vi "Control_stage_event_que.vi"(11 "Stage control":T2={"Up"=FALSE, "Left"=FALSE, "Right"=FALSE, "Down"=FALSE, "Z Down"=FALSE, "Z Up"=FALSE, "X Step Size(um)"=10.0, "Z step size (um)"=10.0, "Y Step Size(um)"=10.0, "Enable x-axis"=TRUE, "Enable y-axis"=TRUE, "Enable z-axis"=TRUE, "Same step size"=TRUE, "Global step size (um)"=10.0, "stop"=FALSE, "Destination"={"X Position"=-23.0, "Y Position"=-18.0, "Z Position"=0.0}, "Move to destination"=FALSE}) -> (10 "Stage position":T1={"X Position"=-23.0, "Y Position"=-18.0, "Z Position"=0.0})   [LabVIEW 2020]
uses:
  typedefs/typedef_stage_control.ctl
  typedefs/typedef_stage_position.ctl
  typedefs/typedef_Z_stack.ctl
  typedefs/Laser_toggles_typedef.ctl
  Global stop DAQ.vi
panel:
  in  "Tab Control":enum32{"Manual setup", "Acquisition", "Debug"}(tab)
  out "FirmwareVersion":string="3.03\r"
  out "Connected":bool=TRUE
  in  "Laser order control":T3={"Laser 488 nm power"=0.0, "Laser 560 nm power"=0.0, "Laser 595 nm power"=0.0, "Laser 642 nm power"=0.0, "Laser 560 order selection"=2, "Laser 595 order selection"=0, "Laser 642 order selection"=0, "Laser 488 order selection"=1} {"Laser 488 order selection" items=["Not active", "1", "2", "3", "4"]; "Laser 642 order selection" items=["Not active", "1", "2", "3", "4"]; "Laser 595 order selection" items=["Not active", "1", "2", "3", "4"]; "Laser 560 order selection" items=["Not active", "1", "2", "3", "4"]; "Laser 642 nm power" min=0.0 max=5.0 scale=0.0..100.0; "Laser 595 nm power" min=0.0 max=5.0 scale=0.0..100.0; "Laser 560 nm power" min=0.0 max=5.0 scale=0.0..100.0; "Laser 488 nm power" min=0.0 max=5.0 scale=0.0..100.0}
  in  "Z-stack":T4={"Acquire Z-stack"=FALSE, "Step size (um)"=0.2, "Number of slices"=10.0, "Progress Bar"=10, "Image acquisition time (ms)"=1000.0, "Flyback time (ms)"=32.0} {"Progress Bar" scale=0.0..100.0}
  in  "Voice coil calibration file":path=path "C:/Users/lpk27/Documents/pan-ASLMsynched/pan-ASLM/Calibration files/newcalibration_voice coil input_25msflyback.txt"
  out "Initial offset between stage and generation":u32
  out "Error out":errorcluster
  out "output cluster":T5
  in  "SPIIPLUSCOM660Lib.IAsyncChannel":refnum<k7>
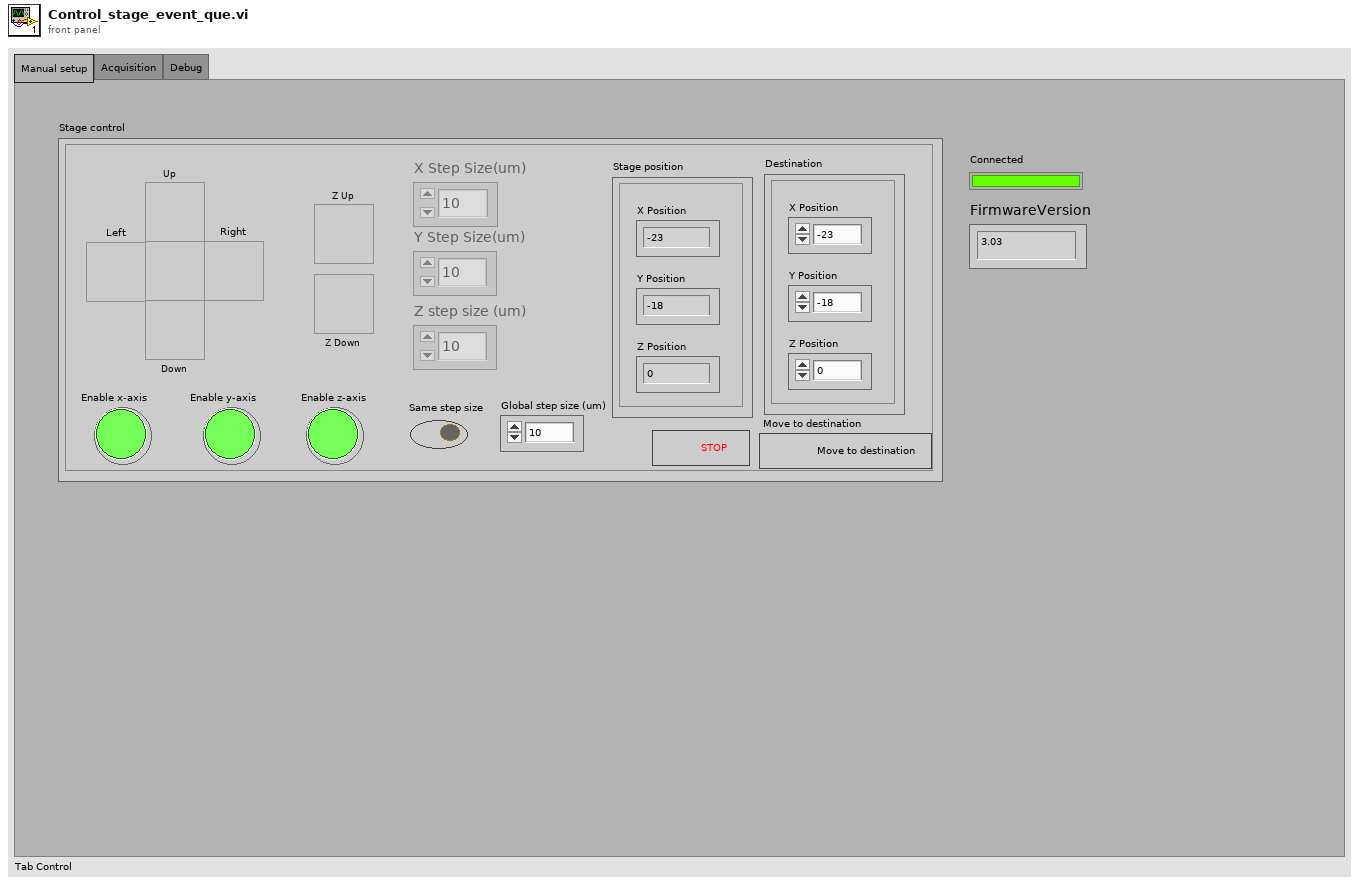
[diagram p1: front panel]
types:
  T1 = typedef "typedef_stage_position.ctl" = cluster{"X Position":dbl, "Y Position":dbl, "Z Position":dbl}
  T2 = typedef "typedef_stage_control.ctl" = cluster{"Up":bool, "Left":bool, "Right":bool, "Down":bool, "Z Down":bool, "Z Up":bool, "X Step Size(um)":dbl, "Z step size (um)":dbl, "Y Step Size(um)":dbl, "Enable x-axis":bool, "Enable y-axis":bool, "Enable z-axis":bool, "Same step size":bool, "Global step size (um)":dbl, "stop":bool, "Destination":T1, "Move to destination":bool}
  T3 = typedef "Laser_toggles_typedef.ctl" = cluster{"Laser 488 nm power":dbl, "Laser 560 nm power":dbl, "Laser 595 nm power":dbl, "Laser 642 nm power":dbl, "Laser 560 order selection":u16, "Laser 595 order selection":u16, "Laser 642 order selection":u16, "Laser 488 order selection":u16}
  T4 = typedef "typedef_Z_stack.ctl" = cluster{"Acquire Z-stack":bool, "Step size (um)":dbl, "Number of slices":dbl, "Progress Bar":u8, "Image acquisition time (ms)":dbl, "Flyback time (ms)":dbl}
  T5 = cluster{"element":string, "reference OUT":refnum<k7>, "error OUT":errorcluster}
  T6 = enum16{"Initialize", "Verify connection", "Running", "Closing"}
  T7 = enum8{"Enabled", "Disabled", "Disabled and Grayed Out"}
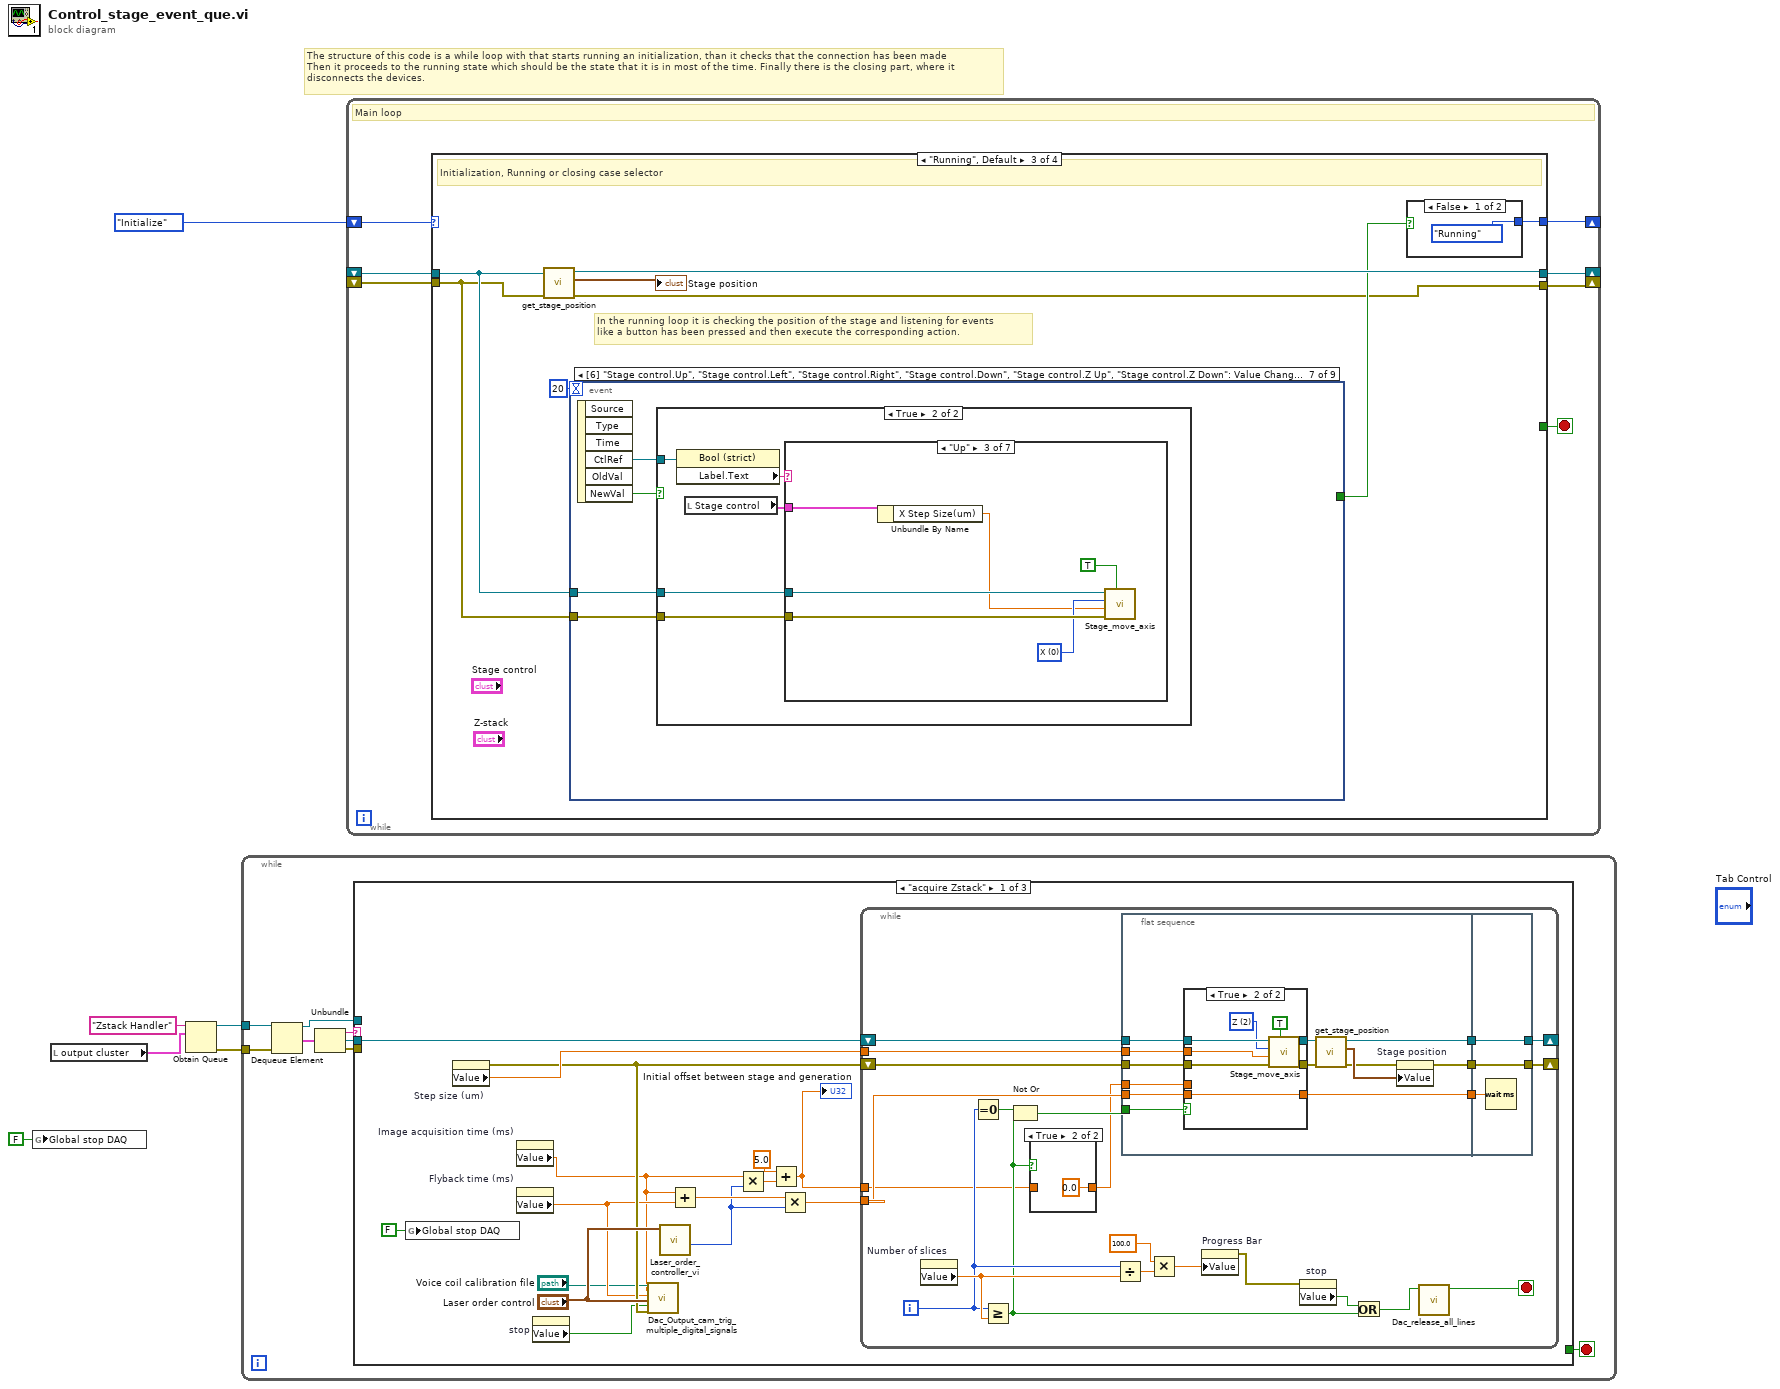
[diagram p0: block diagram]
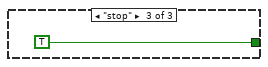
[diagram p5: hidden frame]
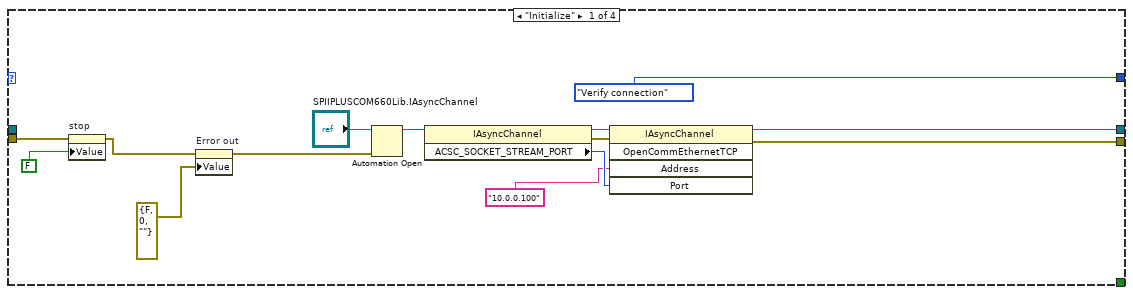
[diagram p6: hidden frame]
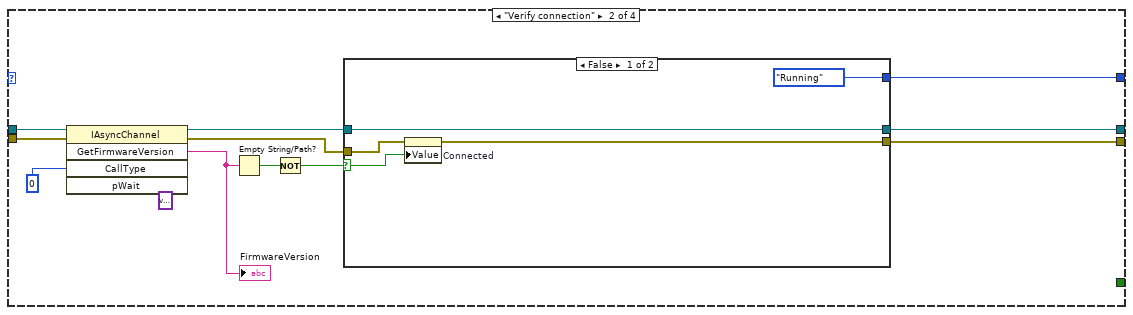
[diagram p7: hidden frame]
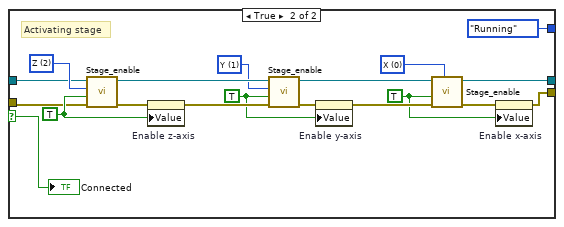
[diagram p8: hidden frame]
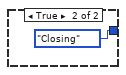
[diagram p9: hidden frame]
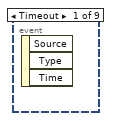
[diagram p10: hidden frame]
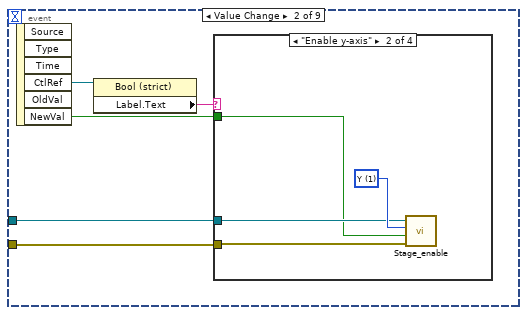
[diagram p11: hidden frame]
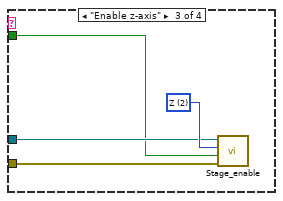
[diagram p13: hidden frame]
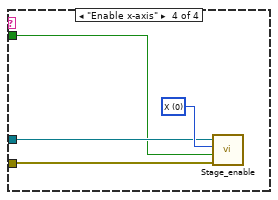
[diagram p14: hidden frame]
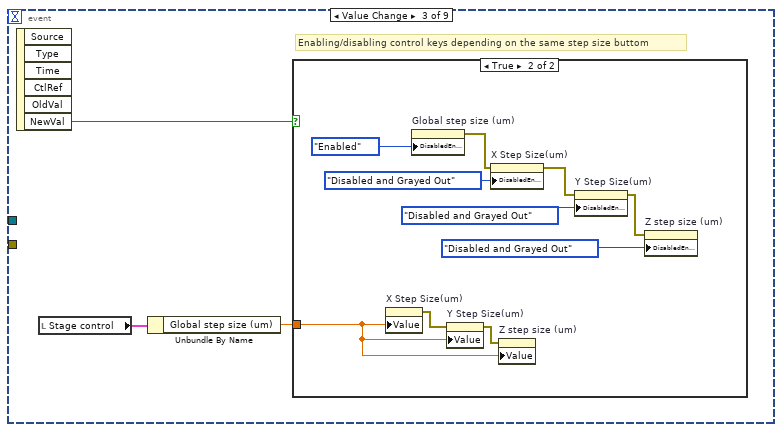
[diagram p15: hidden frame]
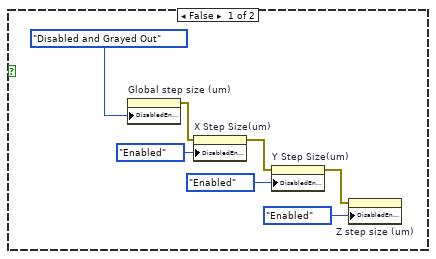
[diagram p16: hidden frame]
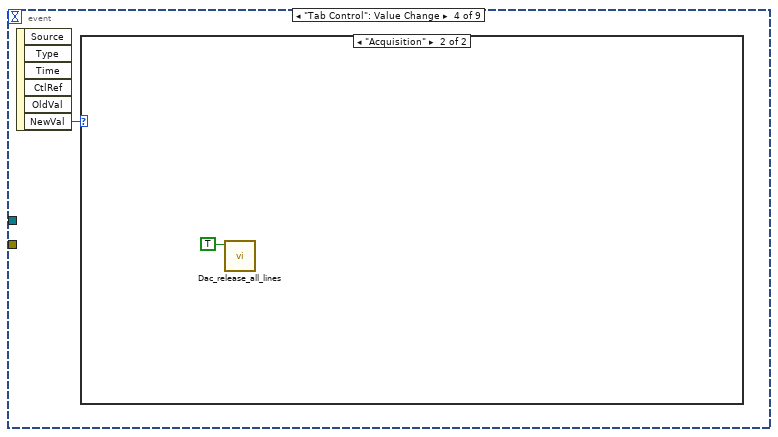
[diagram p17: hidden frame]
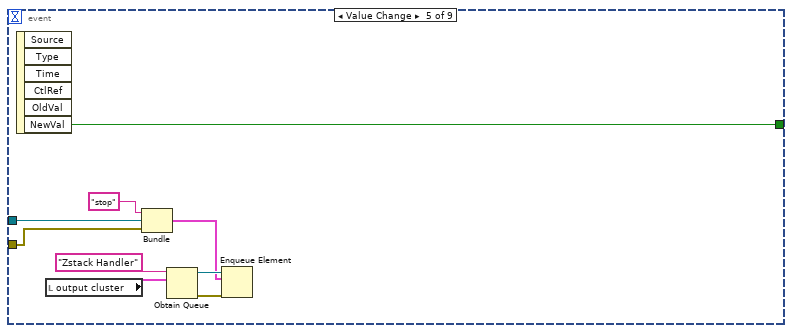
[diagram p19: hidden frame]
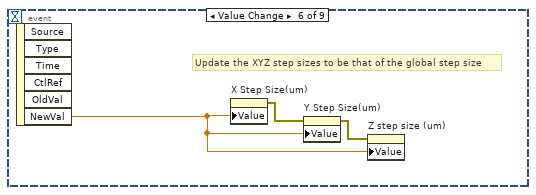
[diagram p20: hidden frame]
diagram:
  # "The structure of this code is a while loop with that starts running an initialization, than it checks that the connection has been made\nThen it proceeds to the running state which should be the state that it is in most of the time. Finally there is the closing part, where it\ndisconnects the devices."
  n1 = global write "Global stop DAQ.vi" "Global stop DAQ"(FALSE ("Global stop DAQ")) -> ()
  n2 = local read "output cluster"() -> (w2:T5)
  n3 = Obtain Queue(name (unnamed)="Zstack Handler", element data type=w2) -> (queue out=w4:refnum<queue>, error out=w3:errorcluster)  [unwired: 3 in, 1 out]
  n4 = while {
    tunnel: w4 -> [w14]
    tunnel: w3 -> [w13]
    stop <- w8 stop-if-true
    n5 = Dequeue Element(queue=w14, error in (no error)=w13) -> (queue out=w7:refnum<queue>, element=w12:T5)  [unwired: 1 in, 2 out]
    n6 = Unbundle(w12) -> ("element"=w11:string, "reference OUT"=w10:refnum<k7>, "error OUT"=w9:errorcluster)
    n7 = case shown="\"acquire Zstack\"" w11 {
      tunnel: w10 -> [w21 _ _]
      tunnel: w9 -> [_ _ _]
      tunnel: [_ _ TRUE] -> w8
      tunnel: w7 -> [_ _ _]
      frame "acquire Zstack" {
        n8 = global write "Global stop DAQ.vi" "Global stop DAQ"(FALSE ("Global stop DAQ")) -> ()
        n9 = property on="Step size (um)" class="DigNum (strict)"() -> (error out=w27:errorcluster, "Value"=w29:dbl)  [unwired: 2 in, 1 out]
        n10 = property on="Image acquisition time (ms)" class="DigNum (strict)"() -> ("Value"=w16:dbl)  [unwired: 2 in, 2 out]
        n11 = property on="Flyback time (ms)" class="DigNum (strict)"() -> ("Value"=w26:dbl)  [unwired: 2 in, 2 out]
        n12 = property on="stop" class="Bool (strict)"() -> ("Value"=w20:bool)  [unwired: 2 in, 2 out]
        n13 = call "Dac_Output_cam_trig_multiple_digital_signals.vi"("File to read"="Voice coil calibration file", "Image acquisition time (ms)"=w16, "Delay between frames"=w26, "Laser Toggles"="Laser order control", "stop"=w20, "error in"=w27) -> ()  [unwired: 13 in, 1 out]
        n14 = call "Laser_order_controller_vi.vi"("Laser Toggles"="Laser order control") -> ("Active lasers"=w18:i16)  [unwired: 8 in, 2 out]
        n15 = Add(x=w16, y=w26) -> (x+y=w25:dbl)
        n16 = Multiply(x=w16, y=w18) -> (x*y=w17:dbl)
        n17 = Add(x=5.0, y=w17) -> (x+y=w15:dbl)
        "Initial offset between stage and generation" <- w15
        n18 = Multiply(x=w25, y=w18) -> (x*y=w23:dbl)
        n19 = while {
          shift-right: [w51] -> _
          shift-left: w21 -> [w52]
          shift-right: [w50] -> _
          shift-left: w27 -> [w38]
          tunnel: w29 -> [w46]
          tunnel: w23 -> [w32]
          tunnel: w15 -> [w31]
          i -> [w37]
          stop <- w41 stop-if-true
          n20 = property on="Number of slices" class="DigNum (strict)"() -> ("Value"=w44:dbl)  [unwired: 2 in, 2 out]
          n21 = Equal To 0?(x=w37) -> (x = 0?=w35:bool)
          n22 = Greater Or Equal?(x=w37, y=w44) -> (x >= y?=w33:bool)
          n23 = Not Or(1:w33, 2:w35) -> (0:w34:bool)
          n24 = case shown="True" w33 {
            tunnel: w31 -> [w53 _]
            tunnel: [w53 0.0] -> w30
            frame False {
            }
            frame True {
            }
          }
          n25 = Divide(x=w37, y=w44) -> (x/y=w48:dbl)
          n26 = flat-sequence {
            tunnel: w52 -> [w67]
            tunnel: w46 -> [w64]
            tunnel: [w66] -> w43
            tunnel: [w65] -> w42
            tunnel: w38 -> [w59]
            tunnel: w34 -> [w58]
            tunnel: w32 -> [w57]
            tunnel: [w56] -> w36
            tunnel: w30 -> [w55]
            tunnel: [w80] -> w50
            tunnel: [w81] -> w51
            tunnel: w43 -> [w81]
            tunnel: w42 -> [w80]
            tunnel: w36 -> [w79]
            frame #0 {
              n27 = case shown="True" w58 {
                tunnel: w67 -> [w70 w78]
                tunnel: w64 -> [_ w77]
                tunnel: [w70 w74] -> w63
                tunnel: [w69 w73] -> w62
                tunnel: w59 -> [w69 w72]
                tunnel: w57 -> [_ w71]
                tunnel: [w68 w71] -> w56
                tunnel: w55 -> [w68 _]
                frame False {
                }
                frame True {
                  w76 = u16 2 items=["X", "Y", "Z"] ("Axes Select")
                  n28 = call "Stage_move_axis.vi"("Direction true means positive increment"=TRUE, "error in (no error)"=w72, "Distance micrometer"=w77, "Axes Select"=w76, "reference IN"=w78) -> ("error OUT"=w73:errorcluster, "reference OUT"=w74:refnum<k7>)  [unwired: 5 in]
                }
              }
              n29 = call "get_stage_position.vi"("error IN"=w62, "reference IN"=w63) -> ("error OUT"=w60:errorcluster, "Stage position OUT"=w61:T1, "reference OUT"=w66:refnum<k7>)  [unwired: 7 in]
              n30 = property on="Stage position" class="Clust (strict)"(error in=w60, "Value"=w61) -> (error out=w65:errorcluster)  [unwired: 1 in, 1 out]
            }
            frame #1 {
              n31 = Wait (ms)(milliseconds to wait=w79) -> ()  [unwired: 1 out]
            }
          }
          n32 = Multiply(x=100.0 ("y"), y=w48) -> (x*y=w45:dbl)
          n33 = property on="Progress Bar" class="Slide (strict)"("Value"=w45) -> (error out=w39:errorcluster)  [unwired: 2 in, 1 out]
          n34 = property on="stop" class="Bool (strict)"(error in=w39) -> ("Value"=w49:bool)  [unwired: 1 in, 2 out]
          n35 = Or(x=w49, y=w33) -> (x .or. y?=w40:bool)
          n36 = call "Dac_release_all_lines.vi"("Release all DAQ lines"=w40) -> ("Finished"=w41:bool)  [unwired: 9 in, 1 out]
        }
      }
      frame Default {
      }
      frame "stop" {
      }
    }
  }
  n37 = while {
    shift-right: [w85] -> _
    shift-left: T6."Initialize" -> [w88]
    shift-right: [w87] -> _
    shift-left: _ -> [w84]
    shift-right: [w86] -> _
    shift-left: _ -> [w83]
    stop <- w89 stop-if-true
    # "Main loop"
    n38 = case shown="\"Running\", Default" w88 {
      tunnel: [_ _ _ TRUE ("NewVal")] -> w89
      tunnel: [w97 w107 w143 _] -> w87
      tunnel: [w96 w105 w140 _] -> w86
      tunnel: [T6."Verify connection" w106 w147 _] -> w85
      tunnel: w84 -> [_ w111 w145 w259]
      tunnel: w83 -> [w93 w110 w144 w258]
      frame "Initialize" {
        n39 = property on="stop" class="Bool (strict)"(error in=w93, "Value"=FALSE) -> (error out=w91:errorcluster)  [unwired: 1 in, 1 out]
        n40 = property on="Error out" class="Clust (strict)"(error in=w91, "Value"=errorcluster {"status"=FALSE, "code"=0, "source"=""} ("Error out")) -> (error out=w90:errorcluster)  [unwired: 1 in, 1 out]
        n41 = Automation Open(error in (no error)=w90, Automation Refnum="SPIIPLUSCOM660Lib.IAsyncChannel") -> (Automation Refnum=w103:refnum<k7>)  [unwired: 2 in, 1 out]
        n42 = property class="IAsyncChannel"(reference=w103) -> (reference out=w102:refnum<k7>, error out=w98:errorcluster, "ACSC_SOCKET_STREAM_PORT"=w100:i32)  [unwired: 1 in]
        n43 = invoke class="IAsyncChannel" method="OpenCommEthernetTCP"(reference=w102, error in=w98, "Address"="10.0.0.100", "Port"=w100) -> (reference out=w97:refnum<k7>, error out=w96:errorcluster)  [unwired: 1 in, 3 out]
      }
      frame "Verify connection" {
        n44 = invoke class="IAsyncChannel" method="GetFirmwareVersion"(reference=w111, error in=w110, "CallType"=u64 0, "pWait"=variant) -> (reference out=w108:refnum<k7>, error out=w104:errorcluster, "GetFirmwareVersion"=w113:string)  [unwired: 1 in, 2 out]
        "FirmwareVersion" <- w113
        n45 = Empty String/Path?(string/path=w113) -> (empty?=w112:bool)
        n46 = Not(x=w112) -> (.not. x?=w109:bool)
        n47 = case shown="False" w109 {
          selector: w109 -> [w120 w139]
          tunnel: w104 -> [w119 w126]
          tunnel: w108 -> [w117 w124]
          tunnel: [w118 w123] -> w105
          tunnel: [w117 w122] -> w107
          tunnel: [T6."Running" T6."Running"] -> w106
          frame False {
            n48 = property on="Connected" class="Bool (strict)"(error in=w119, "Value"=w120) -> (error out=w118:errorcluster)  [unwired: 1 in, 1 out]
          }
          frame True {
            w131 = TRUE ("Boolean")
            w128 = u16 0 items=["X", "Y", "Z"] ("Axes Select")
            w130 = TRUE ("Boolean")
            w127 = u16 1 items=["X", "Y", "Z"] ("Axes Select")
            w129 = TRUE ("Boolean")
            w125 = u16 2 items=["X", "Y", "Z"] ("Axes Select")
            # "Activating stage"
            n49 = call "Stage_enable.vi"("error in (no error)"=w126, "ON=true, OFF = false"=w129, "Axes Select"=w125, "reference"=w124) -> ("error out"=w134:errorcluster, "reference out"=w132:refnum<k7>)  [unwired: 6 in]
            n50 = property on="Enable z-axis" class="Bool (strict)"(error in=w134, "Value"=w129) -> (error out=w135:errorcluster)  [unwired: 1 in, 1 out]
            n51 = call "Stage_enable.vi"("error in (no error)"=w135, "ON=true, OFF = false"=w130, "Axes Select"=w127, "reference"=w132) -> ("error out"=w136:errorcluster, "reference out"=w133:refnum<k7>)  [unwired: 6 in]
            n52 = property on="Enable y-axis" class="Bool (strict)"(error in=w136, "Value"=w130) -> (error out=w137:errorcluster)  [unwired: 1 in, 1 out]
            n53 = call "Stage_enable.vi"("error in (no error)"=w137, "ON=true, OFF = false"=w131, "Axes Select"=w128, "reference"=w133) -> ("error out"=w138:errorcluster, "reference out"=w122:refnum<k7>)  [unwired: 6 in]
            n54 = property on="Enable x-axis" class="Bool (strict)"(error in=w138, "Value"=w131) -> (error out=w123:errorcluster)  [unwired: 1 in, 1 out]
            "Connected" <- w139
          }
        }
      }
      frame "Running", Default {
        # "In the running loop it is checking the position of the stage and listening for events \nlike a button has been pressed and then execute the corresponding action."
        # "Initialization, Running or closing case selector"
        n55 = call "get_stage_position.vi"("error IN"=w144, "reference IN"=w145) -> ("error OUT"=w140:errorcluster, "Stage position OUT"=→"Stage position":T1, "reference OUT"=w143:refnum<k7>)  [unwired: 7 in]
        n56 = event shown="[6] \"Stage control.Up\", \"Stage control.Left\", \"Stage control.Right\", \"Stage control.Down\", \"Stage control.Z Up\", \"Stage control.Z Down\": Value Change" {
          selector: _ -> [_ _ _ _ _ _ _ _ _]
          dyn-events: _ -> [_ _ _ _ _ _ _ _ _]
          timeout: 20 -> [_ _ _ _ _ _ _ _ _]
          tunnel: w145 -> [_ w151 _ _ w191 _ w202 w248 w251]
          tunnel: w144 -> [_ w150 _ _ w190 _ w201 w247 w253]
          tunnel: [_ _ _ _ w197 _ _ _ _] -> w141
          event Timeout {
            n57 = event-data() -> ()  [unwired: 1 in, 3 out]
          }
          event Value Change {
            n58 = event-data() -> ("CtlRef"=w154:refnum<vi>, "NewVal"=w152:bool)  [unwired: 1 in, 4 out]
            n59 = property class="Bool (strict)"(reference=w154) -> ("Label.Text"=w153:string)  [unwired: 1 in, 2 out]
            n60 = case shown="\"Enable y-axis\"" w153 {
              tunnel: w152 -> [_ w155 w159 w163]
              tunnel: w151 -> [_ w156 w161 w165]
              tunnel: w150 -> [_ w157 w160 w164]
              frame Default {
              }
              frame "Enable y-axis" {
                w158 = u16 1 items=["X", "Y", "Z"] ("Axes Select")
                n61 = call "Stage_enable.vi"("error in (no error)"=w157, "ON=true, OFF = false"=w155, "Axes Select"=w158, "reference"=w156) -> ()  [unwired: 6 in, 2 out]
              }
              frame "Enable z-axis" {
                w162 = u16 2 items=["X", "Y", "Z"] ("Axes Select")
                n62 = call "Stage_enable.vi"("error in (no error)"=w160, "ON=true, OFF = false"=w159, "Axes Select"=w162, "reference"=w161) -> ()  [unwired: 6 in, 2 out]
              }
              frame "Enable x-axis" {
                w166 = u16 0 items=["X", "Y", "Z"] ("Axes Select")
                n63 = call "Stage_enable.vi"("error in (no error)"=w164, "ON=true, OFF = false"=w163, "Axes Select"=w166, "reference"=w165) -> ()  [unwired: 6 in, 2 out]
              }
            }
          }
          event Value Change {
            # "Enabling/disabling control keys depending on the same step size buttom"
            n64 = event-data() -> ("NewVal"=w169:bool)  [unwired: 1 in, 5 out]
            n65 = local read "Stage control"() -> (w168:T2)
            n66 = Unbundle By Name(w168) -> ("Global step size (um)"=w167:dbl)
            n67 = case shown="True" w169 {
              tunnel: w167 -> [_ w181]
              frame False {
                n68 = property on="Global step size (um)" class="DigNum (strict)"("DisabledEnum"=T7."Disabled and Grayed Out" ("Disabled")) -> (error out=w170:errorcluster)  [unwired: 2 in, 1 out]
                n69 = property on="X Step Size(um)" class="DigNum (strict)"(error in=w170, "DisabledEnum"=T7."Enabled" ("Disabled")) -> (error out=w174:errorcluster)  [unwired: 1 in, 1 out]
                n70 = property on="Y Step Size(um)" class="DigNum (strict)"(error in=w174, "DisabledEnum"=T7."Enabled" ("Disabled")) -> (error out=w172:errorcluster)  [unwired: 1 in, 1 out]
                n71 = property on="Z step size (um)" class="DigNum (strict)"(error in=w172, "DisabledEnum"=T7."Enabled" ("Disabled")) -> ()  [unwired: 1 in, 2 out]
              }
              frame True {
                n72 = property on="X Step Size(um)" class="DigNum (strict)"("Value"=w181) -> (error out=w180:errorcluster)  [unwired: 2 in, 1 out]
                n73 = property on="Global step size (um)" class="DigNum (strict)"("DisabledEnum"=T7."Enabled" ("Disabled")) -> (error out=w177:errorcluster)  [unwired: 2 in, 1 out]
                n74 = property on="Y Step Size(um)" class="DigNum (strict)"(error in=w180, "Value"=w181) -> (error out=w179:errorcluster)  [unwired: 1 in, 1 out]
                n75 = property on="X Step Size(um)" class="DigNum (strict)"(error in=w177, "DisabledEnum"=T7."Disabled and Grayed Out" ("Disabled")) -> (error out=w184:errorcluster)  [unwired: 1 in, 1 out]
                n76 = property on="Z step size (um)" class="DigNum (strict)"(error in=w179, "Value"=w181) -> ()  [unwired: 1 in, 2 out]
                n77 = property on="Y Step Size(um)" class="DigNum (strict)"(error in=w184, "DisabledEnum"=T7."Disabled and Grayed Out" ("Disabled")) -> (error out=w182:errorcluster)  [unwired: 1 in, 1 out]
                n78 = property on="Z step size (um)" class="DigNum (strict)"(error in=w182, "DisabledEnum"=T7."Disabled and Grayed Out" ("Disabled")) -> ()  [unwired: 1 in, 2 out]
              }
            }
          }
          event "Tab Control": Value Change {
            n79 = event-data() -> ("NewVal"=w187:enum32{"Manual setup", "Acquisition", "Debug"})  [unwired: 1 in, 5 out]
            n80 = case shown="\"Acquisition\"" w187 {
              frame "Manual setup", Default {
              }
              frame "Acquisition" {
                n81 = call "Dac_release_all_lines.vi"("Release all DAQ lines"=TRUE) -> ()  [unwired: 9 in, 2 out]
              }
            }
          }
          event Value Change {
            n82 = event-data() -> ("NewVal"=w197:bool)  [unwired: 1 in, 5 out]
            n83 = local read "output cluster"() -> (w193:T5)
            n84 = Bundle("element"="stop", "reference OUT"=w191, "error OUT"=w190) -> (w189:T5)  [unwired: 1 in]
            n85 = Obtain Queue(name (unnamed)="Zstack Handler", element data type=w193) -> (queue out=w195:refnum<queue>, error out=w194:errorcluster)  [unwired: 3 in, 1 out]
            n86 = Enqueue Element(queue=w195, element=w189, error in (no error)=w194) -> ()  [unwired: 1 in, 3 out]
          }
          event Value Change {
            # "Update the XYZ step sizes to be that of the global step size"
            n87 = event-data() -> ("NewVal"=w200:dbl)  [unwired: 1 in, 5 out]
            n88 = property on="X Step Size(um)" class="DigNum (strict)"("Value"=w200) -> (error out=w199:errorcluster)  [unwired: 2 in, 1 out]
            n89 = property on="Y Step Size(um)" class="DigNum (strict)"(error in=w199, "Value"=w200) -> (error out=w198:errorcluster)  [unwired: 1 in, 1 out]
            n90 = property on="Z step size (um)" class="DigNum (strict)"(error in=w198, "Value"=w200) -> ()  [unwired: 1 in, 2 out]
          }
          event Value Change {
            n91 = event-data() -> ("CtlRef"=w204:refnum<vi>, "NewVal"=w203:bool)  [unwired: 1 in, 4 out]
            n92 = case shown="True" w203 {
              tunnel: w204 -> [_ w209]
              tunnel: w202 -> [_ w206]
              tunnel: w201 -> [_ w205]
              frame False {
              }
              frame True {
                n93 = property class="Bool (strict)"(reference=w209) -> ("Label.Text"=w208:string)  [unwired: 1 in, 2 out]
                n94 = local read "Stage control"() -> (w207:T2)
                n95 = case shown="\"Up\"" w208 {
                  tunnel: w207 -> [w215 w221 w227 w233 w239 w245 _]
                  tunnel: w206 -> [w214 w220 w226 w232 w238 w244 _]
                  tunnel: w205 -> [w213 w219 w225 w231 w237 w243 _]
                  frame "Left" {
                    w211 = u16 1 items=["X", "Y", "Z"] ("Axes Select")
                    n96 = Unbundle By Name(w215) -> ("Y Step Size(um)"=w210:dbl)
                    n97 = call "Stage_move_axis.vi"("Direction true means positive increment"=FALSE, "error in (no error)"=w213, "Distance micrometer"=w210, "Axes Select"=w211, "reference IN"=w214) -> ()  [unwired: 5 in, 2 out]
                  }
                  frame "Right" {
                    w217 = u16 1 items=["X", "Y", "Z"] ("Axes Select")
                    n98 = Unbundle By Name(w221) -> ("Y Step Size(um)"=w216:dbl)
                    n99 = call "Stage_move_axis.vi"("Direction true means positive increment"=TRUE, "error in (no error)"=w219, "Distance micrometer"=w216, "Axes Select"=w217, "reference IN"=w220) -> ()  [unwired: 5 in, 2 out]
                  }
                  frame "Up" {
                    w223 = u16 0 items=["X", "Y", "Z"] ("Axes Select")
                    n100 = Unbundle By Name(w227) -> ("X Step Size(um)"=w222:dbl)
                    n101 = call "Stage_move_axis.vi"("Direction true means positive increment"=TRUE, "error in (no error)"=w225, "Distance micrometer"=w222, "Axes Select"=w223, "reference IN"=w226) -> ()  [unwired: 5 in, 2 out]
                  }
                  frame "Down" {
                    w229 = u16 0 items=["X", "Y", "Z"] ("Axes Select")
                    n102 = Unbundle By Name(w233) -> ("X Step Size(um)"=w228:dbl)
                    n103 = call "Stage_move_axis.vi"("Direction true means positive increment"=FALSE, "error in (no error)"=w231, "Distance micrometer"=w228, "Axes Select"=w229, "reference IN"=w232) -> ()  [unwired: 5 in, 2 out]
                  }
                  frame "Z Up" {
                    w235 = u16 2 items=["X", "Y", "Z"] ("Axes Select")
                    n104 = Unbundle By Name(w239) -> ("Z step size (um)"=w234:dbl)
                    n105 = call "Stage_move_axis.vi"("Direction true means positive increment"=TRUE, "error in (no error)"=w237, "Distance micrometer"=w234, "Axes Select"=w235, "reference IN"=w238) -> ()  [unwired: 5 in, 2 out]
                  }
                  frame "Z Down" {
                    w241 = u16 2 items=["X", "Y", "Z"] ("Axes Select")
                    n106 = Unbundle By Name(w245) -> ("Z step size (um)"=w240:dbl)
                    n107 = call "Stage_move_axis.vi"("Direction true means positive increment"=FALSE, "error in (no error)"=w243, "Distance micrometer"=w240, "Axes Select"=w241, "reference IN"=w244) -> ()  [unwired: 5 in, 2 out]
                  }
                  frame Default {
                  }
                }
              }
            }
          }
          event Value Change {
            n108 = event-data() -> ()  [unwired: 1 in, 6 out]
            n109 = property on="Destination" class="Clust (strict)"(error in=w247) -> (error out=w250:errorcluster, "Value"=w249:T1)  [unwired: 1 in, 1 out]
            n110 = call "Stage_move_to_destination.vi"("error IN"=w250, "Stage position IN"=w249, "reference IN"=w248) -> ("Stage position OUT"=w246:T1)  [unwired: 6 in, 2 out]
            n111 = local write "Stage position"(w246) -> ()
          }
          event Value Change {
            n112 = event-data() -> ()  [unwired: 1 in, 6 out]
            n113 = Bundle("element"="acquire Zstack", "reference OUT"=w251, "error OUT"=w253) -> (w252:T5)  [unwired: 1 in]
            "output cluster" <- w252
            n114 = Obtain Queue(name (unnamed)="Zstack Handler", element data type=w252) -> (queue out=w256:refnum<queue>, error out=w255:errorcluster)  [unwired: 3 in, 1 out]
            n115 = Enqueue Element(queue=w256, element=w252, error in (no error)=w255) -> ()  [unwired: 1 in, 3 out]
          }
        }
        n116 = case shown="False" w141 {
          tunnel: [T6."Running" T6."Closing"] -> w147
          frame False {
          }
          frame True {
          }
        }
      }
      frame "Closing" {
        n117 = local write "Connected"(FALSE ("Connected")) -> ()
        n118 = invoke class="IAsyncChannel" method="CloseComm"(reference=w259, error in=w258) -> (error out=→"Error out":errorcluster)  [unwired: 1 in, 2 out]
      }
    }
  }
